vi "Navigation_Main_r1.3(new math for dist calc).vi"() -> ()   [LabVIEW 2015]
uses:
  <vilib>/myRIO/Instrument Drivers/Onboard IO/PWM/typedefs/PWM Reference.ctl
  <vilib>/myRIO/Common/Instrument Driver Framework/Utilities/typedefs/myRIO Generic Hardware Reference.ctl
  <vilib>/myRIO/Common/Instrument Driver Framework/Utilities/typedefs/Hardware Version Enum.ctl
  <vilib>/myRIO/Common/Instrument Driver Framework/Utilities/typedefs/myRIO v1.0 Reference.ctl
  <vilib>/myRIO/Common/Instrument Driver Framework/Utilities/typedefs/Generic FPGA Reference.ctl
  <vilib>/myRIO/Common/Instrument Driver Framework/myRIO v1.0/PWM/typedefs/PWM Channels Enum.ctl
  <vilib>/myRIO/Instrument Drivers/Onboard IO/PWM/typedefs/PWM Configuration.ctl
  <vilib>/userdefined/High Color/nirio_resource_hc.ctl
  <vilib>/myRIO/Common/Instrument Driver Framework/myRIO v1.0/PWM/vis/myRIO v1.1 Open PWM.vi
  <vilib>/myRIO/Common/Instrument Driver Framework/Utilities/vis/Validate Channels.vi
  <vilib>/myRIO/Common/Instrument Driver Framework/myRIO v1.0/PWM/vis/myRIO v1.0 Reserve PWM.vi
  <vilib>/myRIO/Common/Instrument Driver Framework/myRIO v1.0/PWM/vis/myRIO v1.0 Close PWM.vi
  <vilib>/myRIO/Common/Instrument Driver Framework/myRIO v1.0/PWM/vis/myRIO v1.0 Build MUX Configuration PWM.vi
  <vilib>/myRIO/Common/Instrument Driver Framework/myRIO v1.0/Resource Manager/vis/myRIO v1.0 Reserve Channel List.vi
  <vilib>/myRIO/Common/Instrument Driver Framework/myRIO v1.0/PWM/vis/myRIO v1.0 Unreserve PWM.vi
  <vilib>/myRIO/Common/Instrument Driver Framework/myRIO v1.0/Resource Manager/vis/myRIO v1.0 Create Configuration List.vi
  <vilib>/myRIO/Common/Instrument Driver Framework/myRIO v1.0/Resource Manager/vis/myRIO v1.0 Reserve Channel.vi
  <vilib>/myRIO/Common/Instrument Driver Framework/myRIO v1.0/Resource Manager/vis/myRIO v1.0 Unreserve Channel.vi
  <vilib>/myRIO/Common/Instrument Driver Framework/myRIO v1.0/Resource Manager/vis/myRIO v1.0 Unreserve Channel List.vi
  <vilib>/myRIO/Common/Instrument Driver Framework/myRIO v1.0/Resource Manager/vis/myRIO v1.0 Build Mutex Name.vi
  <vilib>/FPGAPlugInAG/myRIO-1900/niLvFpga_Open_myRIO-1900.vi
  <vilib>/rvi/interface/common/dynamic/niFpgaDynamicAddResources.vi
  <vilib>/myRIO/Common/Instrument Driver Framework/Utilities/vis/FPGA Ref Manager.vi
  <vilib>/Utility/error.llb/Error Cluster From Error Code.vi
  <vilib>/myRIO/Common/Instrument Driver Framework/Utilities/vis/Ref Counter.vi
  <vilib>/rvi/errors/niLvFpgaAdjustHostInterfaceError.vi
  <vilib>/Utility/VariantDataType/GetNumericInfo.vi
  <vilib>/myRIO/Common/Instrument Driver Framework/myRIO v1.0/myRIO v1.1 Open.vi
  <vilib>/myRIO/Common/Instrument Driver Framework/Utilities/vis/IO Manager.vi
  <vilib>/myRIO/Common/Instrument Driver Framework/Utilities/vis/Configuration Manager.vi
  <vilib>/myRIO/Common/Instrument Driver Framework/myRIO v1.0/Resource Manager/vis/myRIO v1.0 Configure IO.vi
  <vilib>/myRIO/Common/Instrument Driver Framework/myRIO v1.0/myRIO v1.0 Close.vi
  <vilib>/myRIO/Common/Instrument Driver Framework/myRIO v1.0/PWM/vis/myRIO v1.0 Write PWM.vi
  <vilib>/myRIO/Common/Instrument Driver Framework/myRIO v1.0/PWM/vis/myRIO v1.0 Shutdown PWM.vi
  <vilib>/rvi/interface/nirviOpenFPGA/nirviOpenFPGA.xnode
  Navi/E/FPGA Bitfiles/NavigationProjec_FPGATarget2_FPGAMainNavigati_PWPHW8gwDxI.lvbitx
  <vilib>/rvi/interface/nirviReadWriteControl/nirviReadWriteControl.xnode
  <vilib>/myRIO/Instrument Drivers/Onboard IO/PWM/vis/myRIO PWM Open.xnode
  <vilib>/myRIO/Instrument Drivers/Onboard IO/PWM/PWM.lvlib
  <vilib>/myRIO/Instrument Drivers/Utilities/Utilities.lvlib
  NiFpgaLv.dll
  <vilib>/rvi/interface/Simulation/niFpgaSimulationCallBeginRW.vi
panel:
  out "Tick Count(mSec) 2":u32 caption="Tick Count(mSec)"
  out "Left Setpoint":dbl
  out "Right Setpoint":dbl
  out "robot desired velocity y component\n u2 (ft/s)":dbl
  out "robot desired velocity x component\n u1 (ft/s)":dbl
  out "Desired Velocity":dbl
  out "Reset X Y":dbl
  out "Scale":dbl=1.0
  out "x traveled":dbl
  out "Omega":dbl format="%.2f"
  out "Phi desired":dbl
  out "v right wheel":dbl
  out "v left wheel":dbl
  out "max v":dbl
  in  "loc_x":dbl
  out "x delta":dbl
  out "x position camera":dbl
  out "encoder step sub vi output":dbl[](array[numeric])
  out "Avg R Dist New":dbl
  out "Avg R Step":dbl
  out "Avg L Dist New":dbl
  out "Avg L Step":dbl
  out "Distance Step":dbl
  in  "Avg R Dist Old":dbl
  in  "Avg L Dist Old":dbl
  out "encoder sub vi input array":dbl[](array[numeric])
  out "x & y position output array":dbl[](array[numeric])
  out "x & y position input array":dbl[](array[numeric])
  out "y traveled new":dbl
  out "y position":dbl
  out "x traveled new":dbl
  out "x position":dbl
  out "phi new":dbl
  in  "x traveled old":dbl
  in  "y traveled old":dbl
  in  "phi old":dbl
  in  "Phi Current":dbl format="%#_13g"
  out "omega and angular velocity calc output array":dbl[](array[numeric])
  out "omega and angular velocity calc input array":dbl[](array[numeric])
  out "Wheel  PID SetPoint input Array":dbl[](array[numeric])
  out "Wheel  PID SetPoint output Array":dbl[](array[numeric])
  in  "Goal Position Y":dbl=5.0
  out "track width(ft)":dbl=4.0
  out "RM Distance (ft)":dbl
  out "RR Distance (ft)":dbl
  out "LF Distance (ft)":dbl
  out "LM Distance (ft)":dbl
  out "RF Distance (ft)":dbl
  out "LR Distance (ft)":dbl
  in  "Start Position Y":dbl=5.0
  in  "Goal Position X":dbl=5.0
  in  "Start Position X":dbl=1.0
  in  "All Stop":bool
  in  "Left Side PID Gains":T1={"proportional gain (Kc)"=0.002, "integral time (Ti, min)"=7e-07, "derivative time (Td, min)"=0.0} {"derivative time (Td, min)" format="%.8f"; "integral time (Ti, min)" format="%.8f"; "proportional gain (Kc)" format="%.8f"}
  in  "Left Side Output Range":cluster{"output high":dbl, "output low":dbl}={"output high"=0.13333, "output low"=-0.13333} {"output low" format="%.5f"; "output high" format="%.5f"}
  in  "Right Side PID Gains":T1={"proportional gain (Kc)"=0.002, "integral time (Ti, min)"=7e-07, "derivative time (Td, min)"=0.0} {"derivative time (Td, min)" format="%.8f"; "integral time (Ti, min)" format="%.8f"; "proportional gain (Kc)" format="%.8f"}
  in  "Right Side Output Range":cluster{"output high":dbl, "output low":dbl}={"output high"=0.13333, "output low"=-0.13333} {"output low" format="%.5f"; "output high" format="%.5f"}
  out "Left PWM":dbl
  out "Right PWM":dbl
  out "LF Rot Velocity (rot/s)":dbl
  out "LM Rot Velocity (rot/s)":dbl
  out "LR Rot Velocity (rot/s)":dbl
  out "RR Rot Velocity (rot/s)":dbl
  out "RM Linear Velocity (rot/s)":dbl
  out "RF Linear Velocity (rot/s)":dbl
  in  "Encoder Reset":bool
  out "SYS.SELECTA":u8 format="%08b"
  out "ENC.B_c.CNTR":i32
  out "ENC.B_b.CNTR":i32
  out "ENC.B_a.CNTR":i32
  out "ENC.A_c.CNTR":i32
  out "ENC.A_b.CNTR":i32
  out "ENC.A_a.CNTR":i32
  out "Current Rot Velocity (rot/s)":T2(graph)
  # "Motor Control Parameters"
  # "Press Go when Start and Goal Are Set"
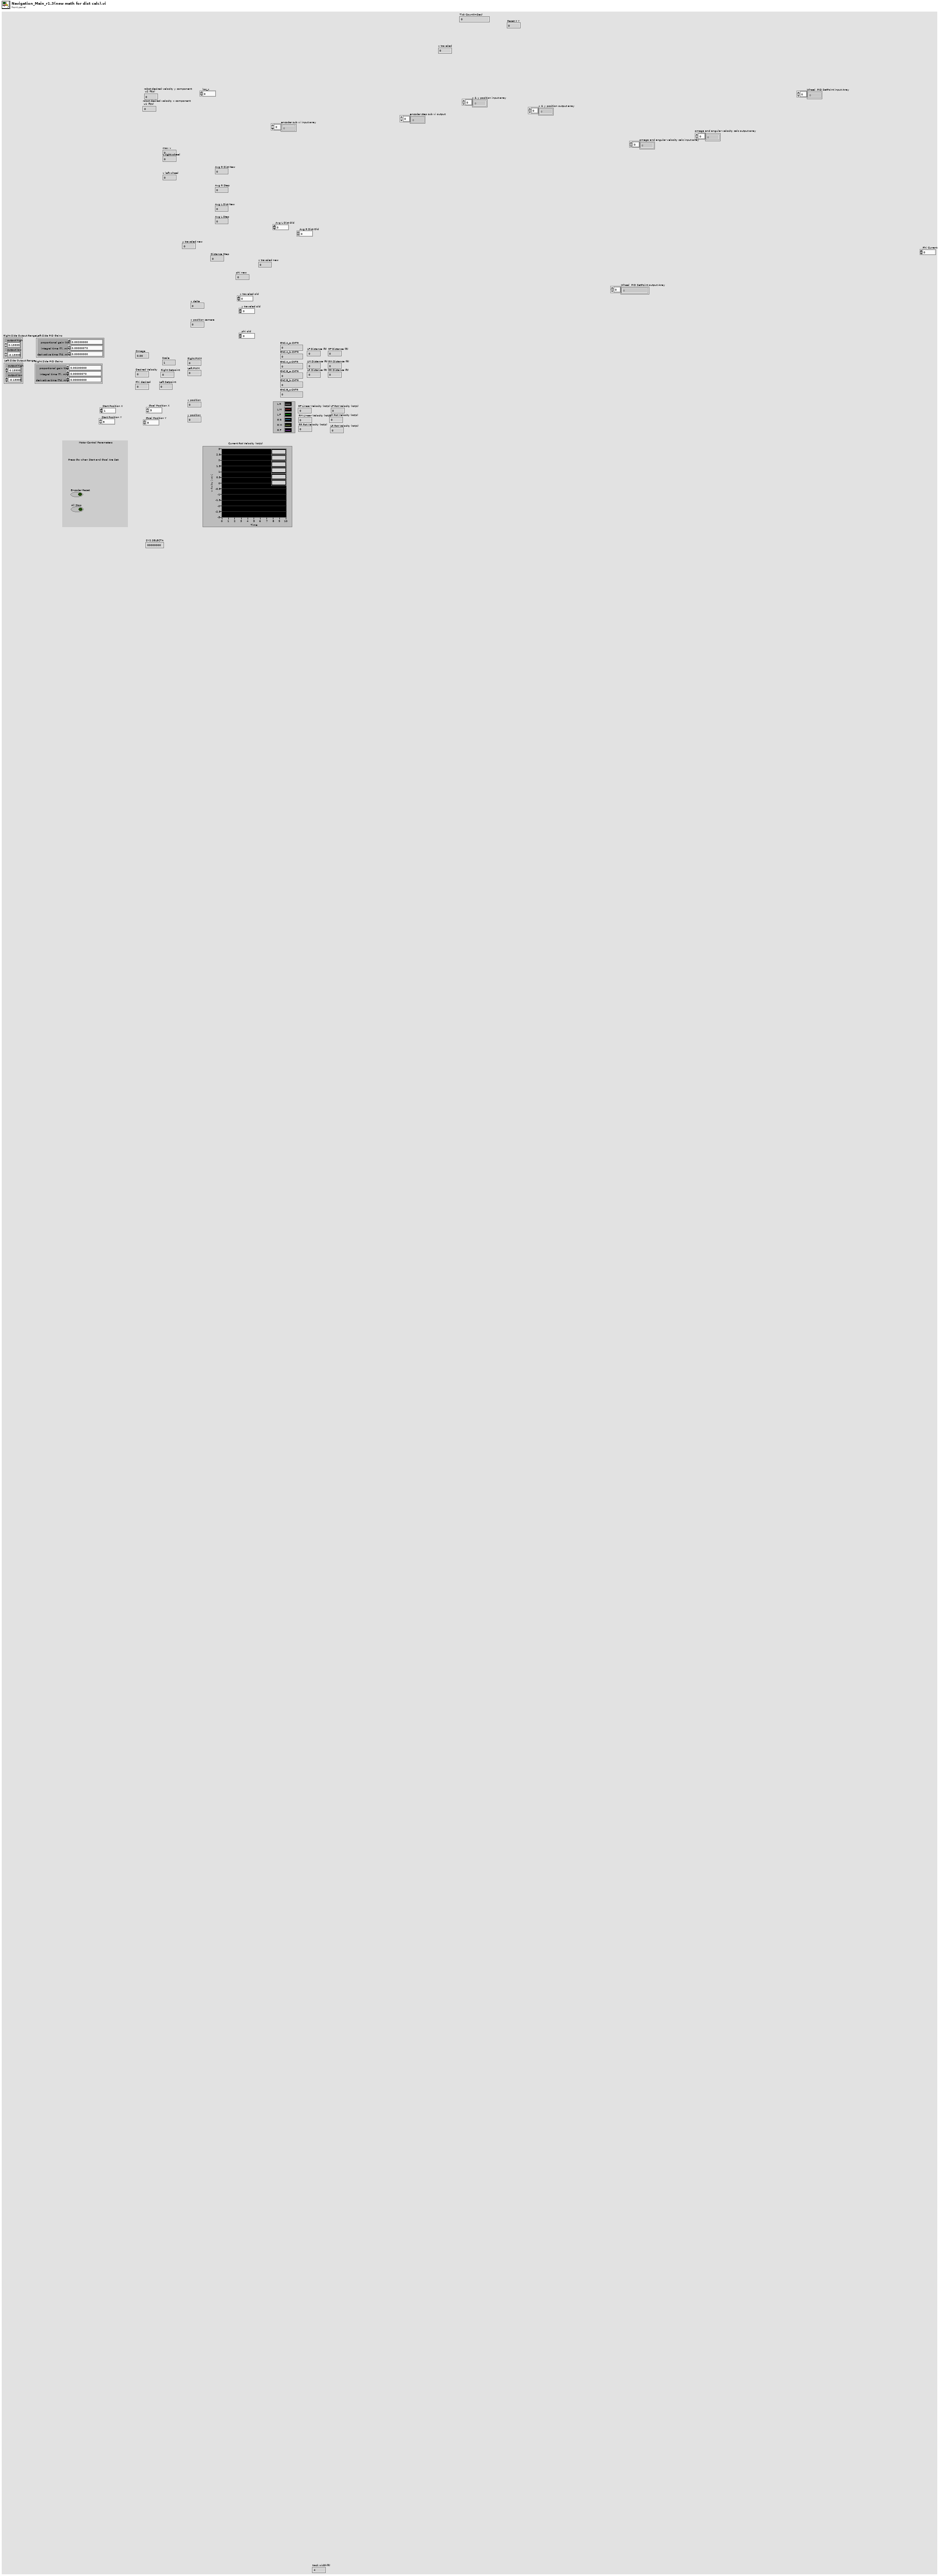
[diagram p1: front panel]
types:
  T1 = cluster{"proportional gain (Kc)":dbl, "integral time (Ti, min)":dbl, "derivative time (Td, min)":dbl}
  T2 = cluster{"Rotational Velocity (RPS)":dbl, "Rotational Velocity (RPS)":dbl, "Rotational Velocity (RPS)":dbl, "Rotational Velocity (RPS)":dbl, "Rotational Velocity (RPS)":dbl, "Rotational Velocity (RPS)":dbl}
  T3 = typedef "nirio_resource_hc.ctl" = tag
  T4 = typedef "Hardware Version Enum.ctl" = enum16{"Unknown", "myRIO-1900", "myRIO-1950", "roboRIO"}
  T5 = typedef "PWM.lvlib/PWM Reference.ctl" = cluster{"myRIO Reference":T6, "PWM Channels Enum":T9, "PWM Configuration":T10}
  T6 = typedef "myRIO Generic Hardware Reference.ctl" = cluster{"myRIO Model":T4, "myRIO Hardware Reference":T7}
  T7 = typedef "myRIO v1.0 Reference.ctl" = cluster{"Generic FPGA Reference":T8, "Allow multiple opens":bool}
  T8 = typedef "Generic FPGA Reference.ctl" = refnum<k20>
  T9 = typedef "PWM Channels Enum.ctl" = enum16{"Not Connected", "C/PWM0", "C/PWM1", "A/PWM0", "A/PWM1", "A/PWM2", "B/PWM0", "B/PWM1", "B/PWM2", "PWM/PWM0", "PWM/PWM1", "PWM/PWM2", "PWM/PWM3", "PWM/PWM4", "PWM/PWM5", "PWM/PWM6", "PWM/PWM7", "PWM/PWM8", "PWM/PWM9"}
  T10 = typedef "PWM.lvlib/PWM Configuration.ctl" = cluster{"Frequency":dbl, "Duty Cycle":dbl}
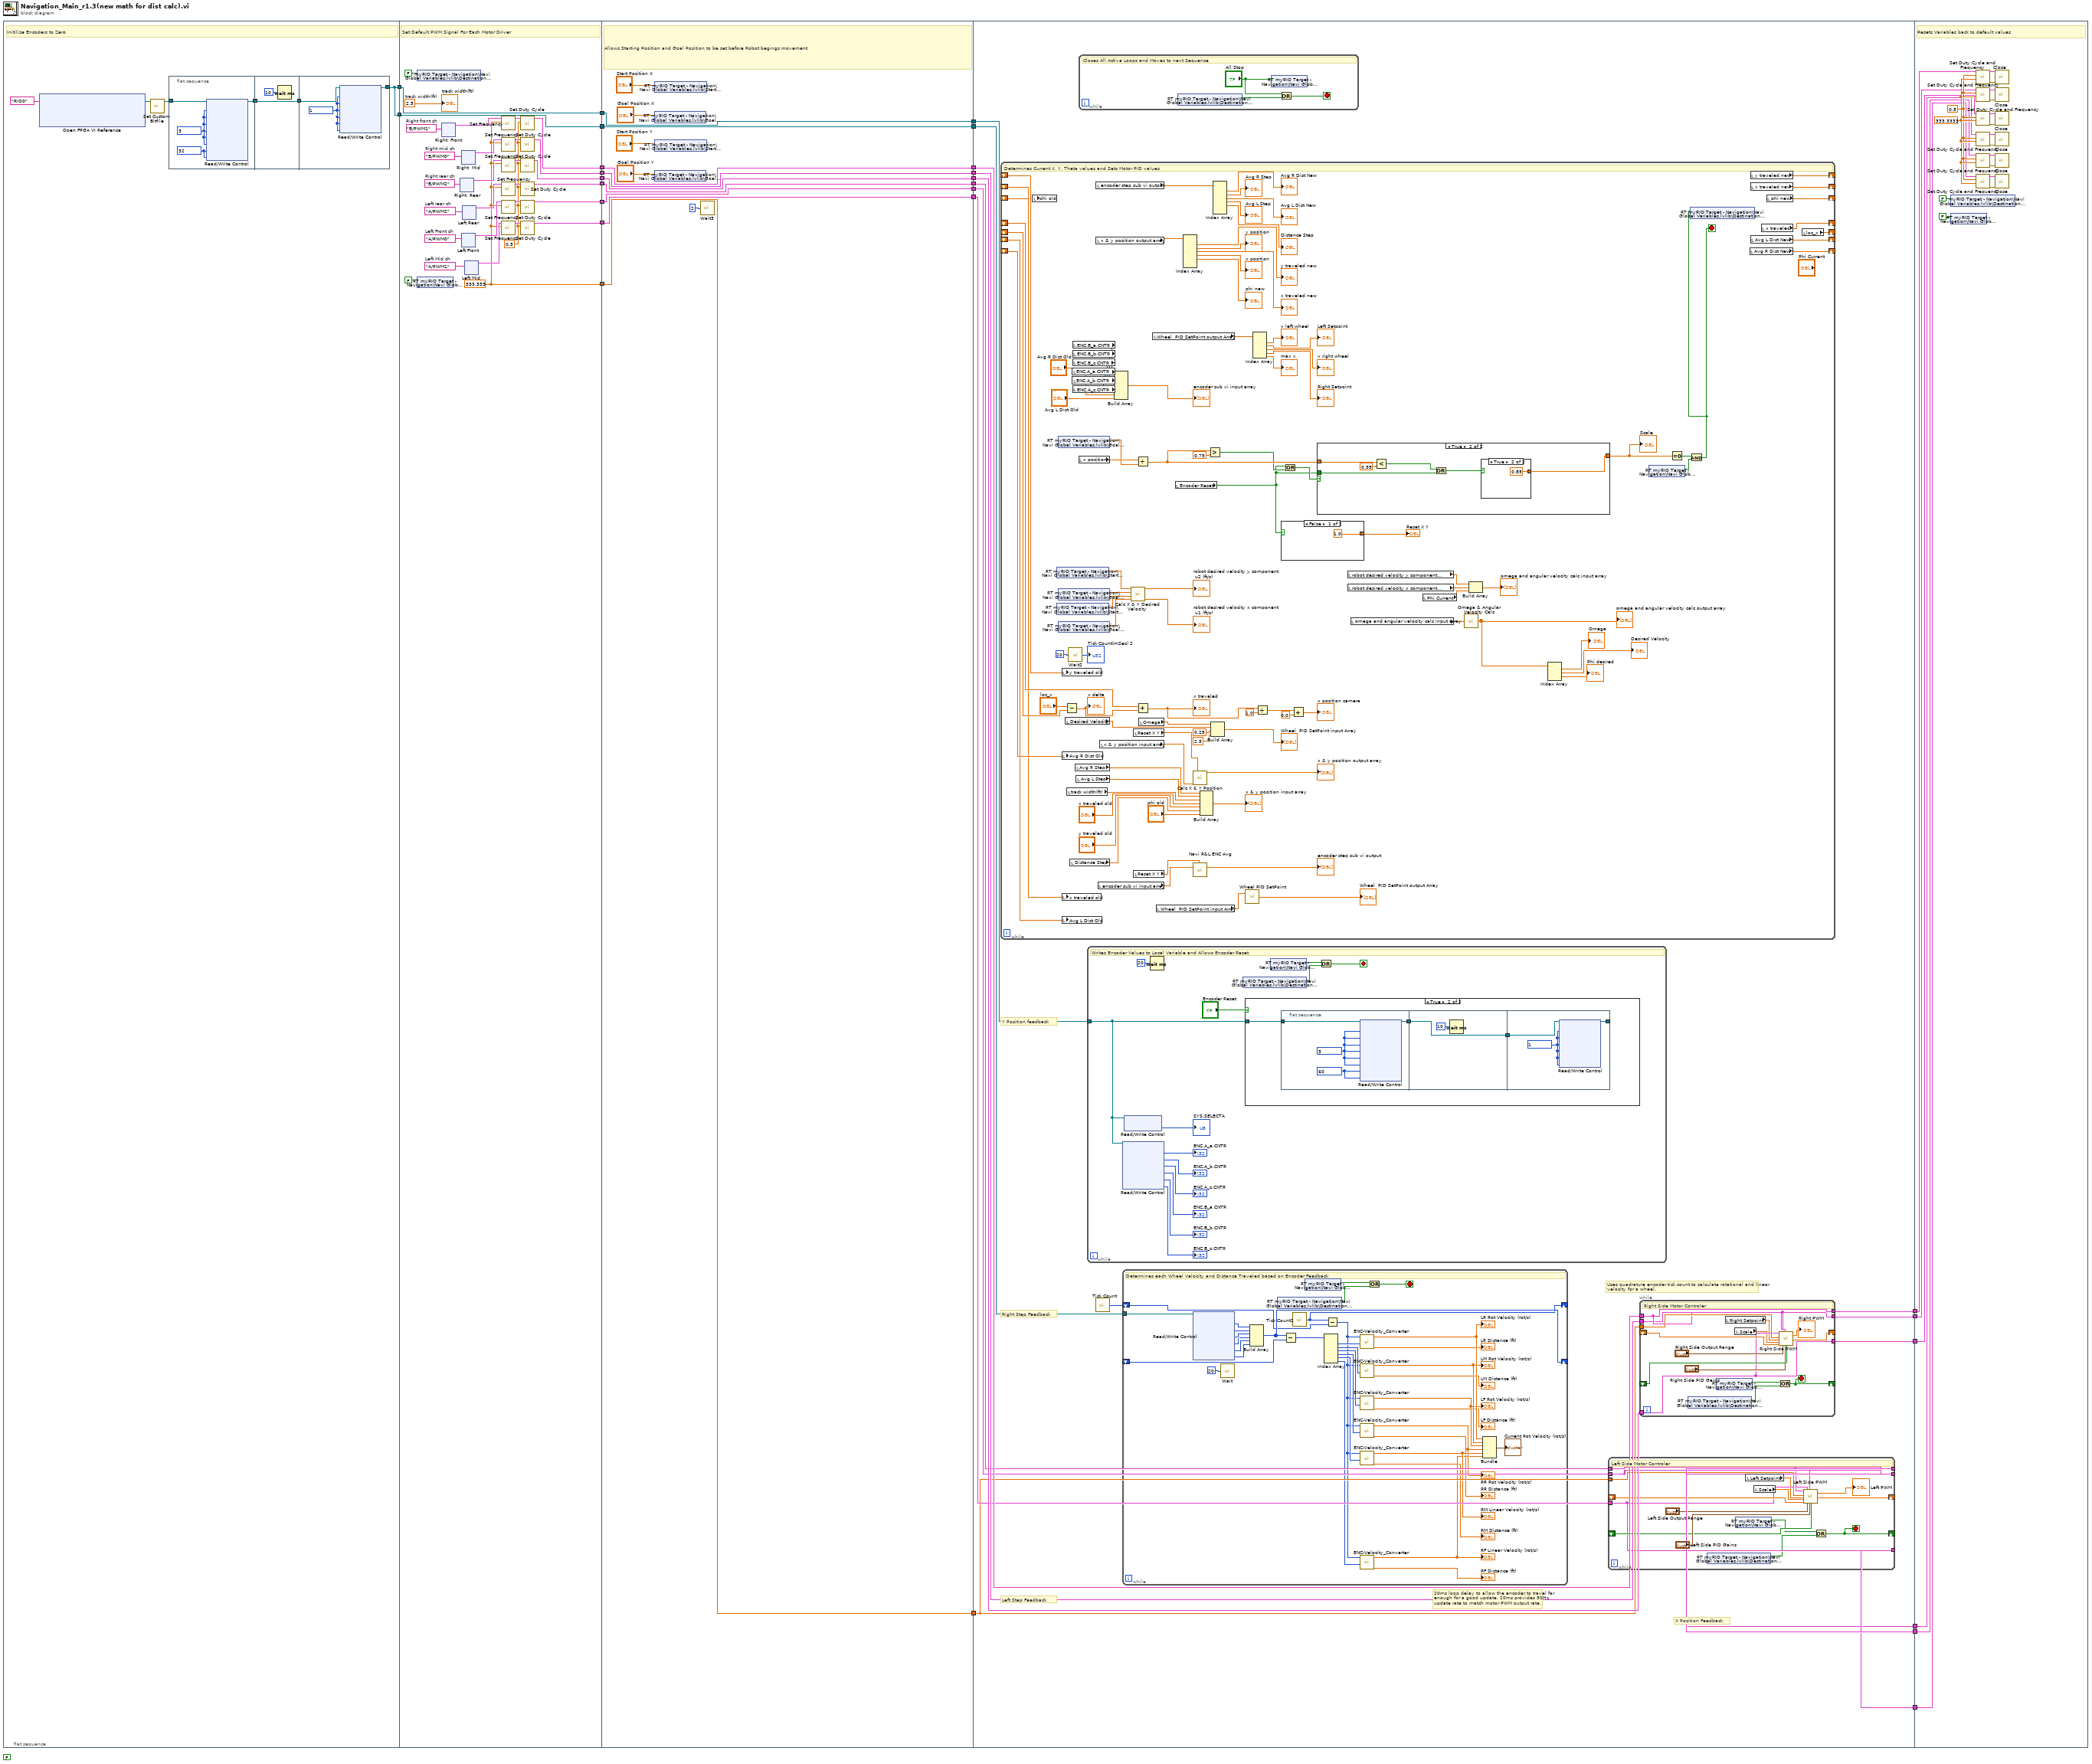
[diagram p0: block diagram]
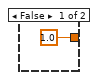
[diagram p2: hidden frame]
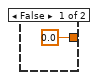
[diagram p3: hidden frame]
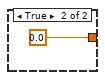
[diagram p4: hidden frame]
diagram:
  (unwired) FALSE ("stop")
  n1 = flat-sequence {
    tunnel: [w29] -> w26
    tunnel: [w29] -> w25
    tunnel: [w60] -> w24
    tunnel: [w55] -> w23
    tunnel: [w51] -> w22
    tunnel: [w50] -> w21
    tunnel: [w49] -> w20
    tunnel: [w48] -> w19
    tunnel: [w47] -> w18
    tunnel: [w46] -> w17
    tunnel: w26 -> [w45]
    tunnel: [w45] -> w16
    tunnel: w25 -> [w46]
    tunnel: w24 -> [w182]
    tunnel: [w182] -> w15
    tunnel: w23 -> [w181]
    tunnel: [w181] -> w14
    tunnel: w22 -> [w180]
    tunnel: [w180] -> w13
    tunnel: w21 -> [w169]
    tunnel: [w169] -> w12
    tunnel: w20 -> [w179]
    tunnel: [w179] -> w11
    tunnel: w19 -> [w178]
    tunnel: [w178] -> w10
    tunnel: w18 -> [w177]
    tunnel: [w177] -> w9
    tunnel: w17 -> [w176]
    tunnel: [w176] -> w8
    tunnel: w16 -> [w175]
    tunnel: [w175] -> w7
    tunnel: w15 -> [w189]
    tunnel: w14 -> [w190]
    tunnel: w13 -> [w195]
    tunnel: w12 -> [w194]
    tunnel: w11 -> [w193]
    tunnel: w10 -> [w192]
    tunnel: w9 -> [w191]
    tunnel: w8 -> [w197]
    tunnel: w7 -> [w196]
    tunnel: [w188] -> w6
    tunnel: [w187] -> w5
    tunnel: [w186] -> w4
    tunnel: [w185] -> w3
    tunnel: [w184] -> w2
    tunnel: [w183] -> w1
    tunnel: w6 -> [w409]
    tunnel: w5 -> [w408]
    tunnel: w4 -> [w407]
    tunnel: w3 -> [w406]
    tunnel: w2 -> [w405]
    tunnel: w1 -> [w404]
    frame #0 {
      # "Initilize Encoders to Zero"
      n2 = xnode "Open FPGA VI Reference"("resource name"=tag "RIO0") -> ("FPGA VI Reference Out"=w28:refnum<k20>)  [unwired: 1 in, 1 out]
      n3 = call <vilib>:"Set Custom Bitfile.vi"("Custom FPGA Reference In"=w28) -> ("Custom FPGA Reference Out"=w30:refnum<k20>)  [unwired: 9 in, 1 out]
      n4 = flat-sequence {
        tunnel: w30 -> [w35]
        tunnel: [w33] -> w32
        tunnel: w32 -> [w37]
        tunnel: [w37] -> w31
        tunnel: w31 -> [w40]
        tunnel: [w39] -> w29
        frame #0 {
          w34 = u8 32 ("SYS.SELECTA")
          w36 = u8 3 ("ENC.B_c.CNFG")
          n5 = xnode "Read/Write Control"("FPGA VI Reference In"=w35, "ENC.A_a.CNFG"=w36, "ENC.A_b.CNFG"=w36, "ENC.A_c.CNFG"=w36, "ENC.B_a.CNFG"=w36, "ENC.B_b.CNFG"=w36, "ENC.B_c.CNFG"=w36, "SYS.SELECTA"=w34, "SYS.SELECTB"=w34) -> ("FPGA VI Reference Out"=w33:refnum<k20>)  [unwired: 1 in, 1 out]
        }
        frame #1 {
          n6 = Wait (ms)(milliseconds to wait=u32 10) -> ()  [unwired: 1 out]
        }
        frame #2 {
          w41 = u8 1 ("ENC.B_c.CNFG")
          n7 = xnode "Read/Write Control"("FPGA VI Reference In"=w40, "ENC.A_a.CNFG"=w41, "ENC.A_b.CNFG"=w41, "ENC.A_c.CNFG"=w41, "ENC.B_a.CNFG"=w41, "ENC.B_b.CNFG"=w41, "ENC.B_c.CNFG"=w41) -> ("FPGA VI Reference Out"=w39:refnum<k20>)  [unwired: 1 in, 1 out]
        }
      }
    }
    frame #1 {
      w42 = 2.5  # track width(ft)
      w52 = 0.5 ("Duty Cycle")
      w60 = 333.333 ("Frequency [Hz]")
      w67 = tag "B/PWM2"  # Right rear ch
      w68 = tag "B/PWM0"  # Right mid ch
      w69 = tag "B/PWM1"  # Right front ch
      w70 = tag "A/PWM2"  # Left rear ch
      w71 = tag "A/PWM0"  # Left Front ch
      w72 = tag "A/PWM1"  # Left Mid ch
      # "Set Default PWM Signal For Each Motor Driver"
      n8 = shared-variable "RT myRIO Target - Navigation\\Navi Global Variables.lvlib\\Destination Reached"(FALSE) -> ()  [unwired: 1 in, 1 out]
      n9 = shared-variable "RT myRIO Target - Navigation\\Navi Global Variables.lvlib\\All Stop"(FALSE) -> ()  [unwired: 1 in, 1 out]
      n10 = xnode "Right  Front"("Channel Name"=w69) -> ("PWM Ref Out"=w63:T5)  [unwired: 2 in, 1 out]
      n11 = xnode "Right  Rear"("Channel Name"=w67) -> ("PWM Ref Out"=w61:T5)  [unwired: 2 in, 1 out]
      n12 = xnode "Right  Mid"("Channel Name"=w68) -> ("PWM Ref Out"=w62:T5)  [unwired: 2 in, 1 out]
      n13 = xnode "Left Front"("Channel Name"=w71) -> ("PWM Ref Out"=w65:T5)  [unwired: 2 in, 1 out]
      n14 = xnode "Left Rear"("Channel Name"=w70) -> ("PWM Ref Out"=w64:T5)  [unwired: 2 in, 1 out]
      n15 = xnode "Left Mid"("Channel Name"=w72) -> ("PWM Ref Out"=w66:T5)  [unwired: 2 in, 1 out]
      n16 = call <vilib>:"Set Frequency.vi"("Frequency [Hz]"=w60, "PWM Ref In"=w63) -> ("PWM Ref Out"=w56:T5)  [unwired: 7 in, 1 out]
      n17 = call <vilib>:"Set Frequency.vi"("Frequency [Hz]"=w60, "PWM Ref In"=w62) -> ("PWM Ref Out"=w57:T5)  [unwired: 7 in, 1 out]
      n18 = call <vilib>:"Set Frequency.vi"("Frequency [Hz]"=w60, "PWM Ref In"=w61) -> ("PWM Ref Out"=w58:T5)  [unwired: 7 in, 1 out]
      n19 = call <vilib>:"Set Frequency.vi"("Frequency [Hz]"=w60, "PWM Ref In"=w64) -> ("PWM Ref Out"=w54:T5)  [unwired: 7 in, 1 out]
      n20 = call <vilib>:"Set Frequency.vi"("Frequency [Hz]"=w60, "PWM Ref In"=w65) -> ("PWM Ref Out"=w53:T5)  [unwired: 7 in, 1 out]
      n21 = call <vilib>:"Set Frequency.vi"("Frequency [Hz]"=w60, "PWM Ref In"=w66) -> ("PWM Ref Out"=w59:T5)  [unwired: 7 in, 1 out]
      n22 = call <vilib>:"Set Duty Cycle.vi"("Duty Cycle"=w52, "PWM Ref In"=w56) -> ("PWM Ref Out"=w51:T5)  [unwired: 7 in, 1 out]
      n23 = call <vilib>:"Set Duty Cycle.vi"("Duty Cycle"=w52, "PWM Ref In"=w57) -> ("PWM Ref Out"=w50:T5)  [unwired: 7 in, 1 out]
      n24 = call <vilib>:"Set Duty Cycle.vi"("Duty Cycle"=w52, "PWM Ref In"=w58) -> ("PWM Ref Out"=w49:T5)  [unwired: 7 in, 1 out]
      n25 = call <vilib>:"Set Duty Cycle.vi"("Duty Cycle"=w52, "PWM Ref In"=w54) -> ("PWM Ref Out"=w55:T5)  [unwired: 7 in, 1 out]
      n26 = call <vilib>:"Set Duty Cycle.vi"("Duty Cycle"=w52, "PWM Ref In"=w53) -> ("PWM Ref Out"=w48:T5)  [unwired: 7 in, 1 out]
      n27 = call <vilib>:"Set Duty Cycle.vi"("Duty Cycle"=w52, "PWM Ref In"=w59) -> ("PWM Ref Out"=w47:T5)  [unwired: 7 in, 1 out]
      "track width(ft)" <- w42
    }
    frame #2 {
      # "Allows Starting Position and Goal Position to be set before Robot begings movement"
      n28 = shared-variable "RT myRIO Target - Navigation\\Navi Global Variables.lvlib\\Start Position X"("Start Position X") -> ()  [unwired: 1 in, 1 out]
      n29 = shared-variable "RT myRIO Target - Navigation\\Navi Global Variables.lvlib\\Goal Position X"("Goal Position X") -> ()  [unwired: 1 in, 1 out]
      n30 = shared-variable "RT myRIO Target - Navigation\\Navi Global Variables.lvlib\\Start Position Y"("Start Position Y") -> ()  [unwired: 1 in, 1 out]
      n31 = shared-variable "RT myRIO Target - Navigation\\Navi Global Variables.lvlib\\Goal Position Y"("Goal Position Y") -> ()  [unwired: 1 in, 1 out]
      n32 = call "Wait3"("Count(mSec)"=u32 2) -> ()  [unwired: 1 out]
    }
    frame #3 {
      # "Left Step Feedback"
      # "Y Position feedback"
      # "Right Step Feedback"
      # "X Position Feedback"
      # "Uses quadrature encoder tick count to calculate rotational and linear velocity for a wheel."
      # "20ms loop delay to allow the encoder to travel far enough for a good update. 20ms provides 50Hz update rate to match motor PWM output rate."
      n33 = while {
        shift-right: [w278] -> _
        shift-left: _ -> [w279]
        shift-right: [w275] -> _
        shift-left: _ -> [w276]
        shift-right: [w238] -> _
        shift-left: _ -> [w260]
        shift-right: [w239] -> _
        shift-left: _ -> [w261]
        shift-right: [w235] -> _
        shift-left: _ -> [w229]
        shift-right: [w236] -> _
        shift-left: _ -> [w230]
        shift-right: [w237] -> _
        shift-left: _ -> [w228]
        stop <- w200 stop-if-true
        # "Determines Current X, Y, Theta values and Sets Motor PID values"
        n34 = local write "phi old"(w228) -> ()
        n35 = shared-variable "RT myRIO Target - Navigation\\Navi Global Variables.lvlib\\Start Position Y"() -> (w293:dbl)  [unwired: 1 in, 1 out]
        n36 = shared-variable "RT myRIO Target - Navigation\\Navi Global Variables.lvlib\\Start Position X"() -> (w291:dbl)  [unwired: 1 in, 1 out]
        n37 = shared-variable "RT myRIO Target - Navigation\\Navi Global Variables.lvlib\\Goal Position X"() -> (w285:dbl)  [unwired: 1 in, 1 out]
        n38 = shared-variable "RT myRIO Target - Navigation\\Navi Global Variables.lvlib\\Goal Position Y"() -> (w292:dbl)  [unwired: 1 in, 1 out]
        n39 = shared-variable "RT myRIO Target - Navigation\\Navi Global Variables.lvlib\\Goal Position X"() -> (w290:dbl)  [unwired: 1 in, 1 out]
        n40 = local write "y traveled old"(w229) -> ()
        n41 = local write "Avg R Dist Old"(w261) -> ()
        n42 = local write "x traveled old"(w230) -> ()
        n43 = local write "Avg L Dist Old"(w260) -> ()
        n44 = Subtract(x="loc_x", y=w279) -> (x-y=w277:dbl)
        "x delta" <- w277
        n45 = local read "Desired Velocity"() -> (w217:dbl)
        n46 = local read "track width(ft)"() -> (w248:dbl)
        n47 = call "Wait2"("Count(mSec)"=u32 20) -> ("Tick Count(mSec)"=→"Tick Count(mSec) 2":u32)
        n48 = local read "Distance Step"() -> (w232:dbl)
        n49 = local read "ENC.A_a.CNTR"() -> (w254:i32)
        n50 = local read "ENC.A_b.CNTR"() -> (w255:i32)
        n51 = local read "ENC.B_a.CNTR"() -> (w251:i32)
        n52 = local read "ENC.B_b.CNTR"() -> (w252:i32)
        n53 = local read "ENC.B_c.CNTR"() -> (w253:i32)
        n54 = local read "ENC.A_c.CNTR"() -> (w256:i32)
        n55 = local read "Avg R Step"() -> (w250:dbl)
        n56 = local read "Avg L Step"() -> (w249:dbl)
        n57 = local read "x position"() -> (w204:dbl)
        n58 = local read "encoder step sub vi output"() -> (w264:dbl[])
        n59 = local read "x & y position output array"() -> (w243:dbl[])
        n60 = local read "encoder sub vi input array"() -> (w269:dbl[])
        n61 = local read "x & y position input array"() -> (w227:dbl[])
        n62 = Build Array(w251, w252, w253, w254, w255, w256, "Avg R Dist Old", "Avg L Dist Old") -> (→"encoder sub vi input array":dbl[])
        n63 = call "Calc X & Y Desired Velocity.vi"("x goal"=w290, "x start"=w291, "Y Goal"=w292, "Y Position"=w293) -> ("robot desired velocity x component\n u1 (ft/s)"=→"robot desired velocity x component\n u1 (ft/s)":dbl, "robot desired velocity y component\n u2 (ft/s)"=→"robot desired velocity y component\n u2 (ft/s)":dbl)  [unwired: 6 in]
        n64 = local read "Reset X Y"() -> (w226:dbl)
        n65 = local read "Reset X Y"() -> (w270:dbl)
        n66 = Divide(x=w204, y=w285) -> (x/y=w286:dbl)
        n67 = Add(x=w276, y=w277) -> (x+y=w274:dbl)
        "x traveled" <- w274
        n68 = local read "Omega"() -> (w216:dbl)
        n69 = local read "Wheel  PID SetPoint output Array"() -> (w210:dbl[])
        n70 = local read "Wheel  PID SetPoint input Array"() -> (w212:dbl[])
        n71 = local read "Encoder Reset"() -> (w280:bool)
        n72 = Index Array(array=w243) -> (element #1=→"y traveled new":dbl, element #2=→"y position":dbl, element #3=→"x traveled new":dbl, element #4=→"x position":dbl, element #5=→"phi new":dbl)  [unwired: 7 in, 2 out]
        n73 = call "Calc X & Y Position.vi"("x & y position input array"=w227, "Reset X Y"=w226) -> ("y & x traveled output array"=→"x & y position output array":dbl[])  [unwired: 16 in, 1 out]
        n74 = call "Navi R&L ENC Avg.vi"("encoder step sub vi input"=w269, "Reset X Y"=w270) -> ("encoder step sub vi output"=→"encoder step sub vi output":dbl[])  [unwired: 17 in]
        n75 = Build Array(w250, w249, w248, "x traveled old", "y traveled old", w232, "phi old") -> (→"x & y position input array":dbl[])
        n76 = Greater?(x=w286, y=0.75) -> (0:w281:bool)
        n77 = Build Array(w216, w217, 0.25 ("element"), 2.5 ("element")) -> (→"Wheel  PID SetPoint input Array":dbl[])
        n78 = Index Array(array=w264) -> (element #1=→"Avg R Dist New":dbl, element #2=→"Avg R Step":dbl, element #3=→"Avg L Dist New":dbl, element #4=→"Avg L Step":dbl, element #5=→"Distance Step":dbl)  [unwired: 7 in, 2 out]
        n79 = call "Wheel PID SetPoint.vi"("Wheel  PID SetPoint Input Array"=w212) -> ("Wheel  PID SetPoint output Array"=→"Wheel  PID SetPoint output Array":dbl[])  [unwired: 1 in]
        n80 = Index Array(array=w210) -> (element #1=→"v left wheel":dbl, element #2=→"Left Setpoint":dbl, element #3=→"v right wheel":dbl, element #4=→"Right Setpoint":dbl, element #5=→"max v":dbl)  [unwired: 5 in]
        n81 = Divide(x=w274, y=1.0) -> (x/y=w272:dbl)
        n82 = case shown="False" w280 {
          tunnel: [1.0 0.0] -> w287
          frame False {
          }
          frame True {
          }
        }
        "Reset X Y" <- w287
        n83 = Or(x=w280, y=w281) -> (x .or. y?=w282:bool)
        n84 = Add(x=w272, y=0.0) -> (x+y=→"x position camera":dbl)
        n85 = case shown="True" w282 {
          tunnel: w286 -> [_ w303]
          tunnel: [1.0 w300] -> w283
          tunnel: w280 -> [_ w298]
          frame False {
          }
          frame True {
            n86 = Less?(x=w303, y=0.95) -> (x < y?=w301:bool)
            n87 = Or(x=w301, y=w298) -> (x .or. y?=w299:bool)
            n88 = case shown="True" w299 {
              tunnel: [0.0 0.85] -> w300
              frame False {
              }
              frame True {
              }
            }
          }
        }
        "Scale" <- w283
        n89 = local read "robot desired velocity y component\n u2 (ft/s)"() -> (w222:dbl)
        n90 = local read "robot desired velocity x component\n u1 (ft/s)"() -> (w224:dbl)
        n91 = local read "omega and angular velocity calc input array"() -> (w225:dbl[])
        n92 = local read "Phi Current"() -> (w223:dbl)
        n93 = call "Omega & Angular Velocity Calc.vi"("omega and angular velocity calc input array"=w225) -> ("omega and angular velocity calc output array"=w199:dbl[])  [unwired: 4 in]
        "omega and angular velocity calc output array" <- w199
        n94 = Build Array(w222, w224, w223) -> (→"omega and angular velocity calc input array":dbl[])
        n95 = Index Array(array=w199) -> (element #1=→"Omega":dbl, element #2=→"Desired Velocity":dbl, element #3=→"Phi desired":dbl)  [unwired: 3 in]
        n96 = shared-variable "RT myRIO Target - Navigation\\Navi Global Variables.lvlib\\All Stop"() -> (w294:bool)  [unwired: 1 in, 1 out]
        n97 = Equal To 0?(x=w283) -> (x = 0?=w201:bool)
        n98 = And(x=w201, y=w294) -> (x .and. y?=w200:bool)
        n99 = shared-variable "RT myRIO Target - Navigation\\Navi Global Variables.lvlib\\Destination Reached"(w200) -> ()  [unwired: 1 in, 1 out]
        n100 = local read "Avg R Dist New"() -> (w239:dbl)
        n101 = local read "y traveled new"() -> (w235:dbl)
        n102 = local read "x traveled new"() -> (w236:dbl)
        n103 = local read "Avg L Dist New"() -> (w238:dbl)
        n104 = local read "x traveled"() -> (w275:dbl)
        n105 = local read "phi new"() -> (w237:dbl)
        n106 = local read "loc_x"() -> (w278:dbl)
      }
      n107 = while {
        stop <- w310 stop-if-true
        # "Closes All Active Loops and Moves to next Sequence"
        n108 = shared-variable "RT myRIO Target - Navigation\\Navi Global Variables.lvlib\\Destination Reached"() -> (w308:bool)  [unwired: 1 in, 1 out]
        n109 = shared-variable "RT myRIO Target - Navigation\\Navi Global Variables.lvlib\\All Stop"("All Stop") -> ()  [unwired: 1 in, 1 out]
        n110 = Or(x="All Stop", y=w308) -> (x .or. y?=w310:bool)
      }
      n111 = while {
        tunnel: w197 -> [w344]
        stop <- w341 stop-if-true
        # "Writes Encoder Values to Local Variable and Allows Encoder Reset"
        n112 = xnode "Read/Write Control"("FPGA VI Reference In"=w344) -> ("ENC.A_a.CNTR"=→"ENC.A_a.CNTR":u32, "ENC.A_b.CNTR"=→"ENC.A_b.CNTR":u32, "ENC.A_c.CNTR"=→"ENC.A_c.CNTR":u32, "ENC.B_a.CNTR"=→"ENC.B_a.CNTR":u32, "ENC.B_b.CNTR"=→"ENC.B_b.CNTR":u32, "ENC.B_c.CNTR"=→"ENC.B_c.CNTR":u32)  [unwired: 1 in, 2 out]
        n113 = xnode "Read/Write Control"("FPGA VI Reference In"=w344) -> ("SYS.SELECTA"=→"SYS.SELECTA":u8)  [unwired: 1 in, 2 out]
        n114 = Wait (ms)(milliseconds to wait=u32 20) -> ()  [unwired: 1 out]
        n115 = shared-variable "RT myRIO Target - Navigation\\Navi Global Variables.lvlib\\Destination Reached"() -> (w343:bool)  [unwired: 1 in, 1 out]
        n116 = case shown="True" "Encoder Reset" {
          tunnel: w344 -> [_ w354]
          frame False {
          }
          frame True {
            n117 = flat-sequence {
              tunnel: w354 -> [w359]
              tunnel: [w357] -> w356
              tunnel: w356 -> [w361]
              tunnel: [w361] -> w355
              tunnel: w355 -> [w364]
              tunnel: [w363] -> _
              frame #0 {
                w358 = u8 60 ("SYS.SELECTA")
                w360 = u8 3 ("ENC.B_c.CNFG")
                n118 = xnode "Read/Write Control"("FPGA VI Reference In"=w359, "ENC.A_a.CNFG"=w360, "ENC.A_b.CNFG"=w360, "ENC.A_c.CNFG"=w360, "ENC.B_a.CNFG"=w360, "ENC.B_b.CNFG"=w360, "ENC.B_c.CNFG"=w360, "SYS.SELECTA"=w358, "SYS.SELECTB"=w358) -> ("FPGA VI Reference Out"=w357:refnum<k20>)  [unwired: 1 in, 1 out]
              }
              frame #1 {
                n119 = Wait (ms)(milliseconds to wait=u32 10) -> ()  [unwired: 1 out]
              }
              frame #2 {
                w365 = u8 1 ("ENC.B_c.CNFG")
                n120 = xnode "Read/Write Control"("FPGA VI Reference In"=w364, "ENC.A_a.CNFG"=w365, "ENC.A_b.CNFG"=w365, "ENC.A_c.CNFG"=w365, "ENC.B_a.CNFG"=w365, "ENC.B_b.CNFG"=w365, "ENC.B_c.CNFG"=w365) -> ("FPGA VI Reference Out"=w363:refnum<k20>)  [unwired: 1 in, 1 out]
              }
            }
          }
        }
        n121 = shared-variable "RT myRIO Target - Navigation\\Navi Global Variables.lvlib\\All Stop"() -> (w342:bool)  [unwired: 1 in, 1 out]
        n122 = Or(x=w342, y=w343) -> (x .or. y?=w341:bool)
      }
      n123 = call "Tick Count"() -> ("Tick Count(uSec)"=w198:u32)
      n124 = while {
        shift-right: [w393] -> _
        shift-left: _ -> [w392]
        shift-right: [w390] -> _
        shift-left: w198 -> [w389]
        tunnel: w196 -> [w400]
        stop <- w385 stop-if-true
        # "Determines each Wheel Velocity and Distance Traveled based on Encoder Feedback"
        n125 = xnode "Read/Write Control"("FPGA VI Reference In"=w400) -> ("ENC.A_a.CNTR"=w399:u32, "ENC.A_b.CNTR"=w398:u32, "ENC.A_c.CNTR"=w397:u32, "ENC.B_a.CNTR"=w396:u32, "ENC.B_b.CNTR"=w395:u32, "ENC.B_c.CNTR"=w394:u32)  [unwired: 1 in, 2 out]
        n126 = call "Wait"("Count(mSec)"=u32 20) -> ()  [unwired: 1 out]
        n127 = Build Array(w399, w398, w397, w396, w395, w394) -> (w393:u32[])
        n128 = shared-variable "RT myRIO Target - Navigation\\Navi Global Variables.lvlib\\Destination Reached"() -> (w387:bool)  [unwired: 1 in, 1 out]
        n129 = Subtract(x=w393, y=w392) -> (x-y=w391:u32[])
        n130 = call "Tick Count2"() -> ("Tick Count(uSec)"=w390:u32)
        n131 = shared-variable "RT myRIO Target - Navigation\\Navi Global Variables.lvlib\\All Stop"() -> (w386:bool)  [unwired: 1 in, 1 out]
        n132 = Index Array(array=w391) -> (element #1=w384:u32, element #2=w381:u32, element #3=w379:u32, element #4=w377:u32, element #5=w375:u32, element #6=w372:u32)  [unwired: 6 in]
        n133 = Subtract(x=w390, y=w389) -> (x-y=w373:u32)
        n134 = call "ENC-Velocity_Converter.vi"("delta  Encoder Count"=w384, "dt (uSec)"=w373) -> ("Distance (ft)"=→"LR Distance (ft)":dbl, "Rotational Velocity (RPS)"=w383:dbl)  [unwired: 7 in, 1 out]
        "LR Rot Velocity (rot/s)" <- w383
        n135 = call "ENC-Velocity_Converter.vi"("delta  Encoder Count"=w381, "dt (uSec)"=w373) -> ("Distance (ft)"=→"LM Distance (ft)":dbl, "Rotational Velocity (RPS)"=w382:dbl)  [unwired: 7 in, 1 out]
        "LM Rot Velocity (rot/s)" <- w382
        n136 = call "ENC-Velocity_Converter.vi"("delta  Encoder Count"=w379, "dt (uSec)"=w373) -> ("Distance (ft)"=→"LF Distance (ft)":dbl, "Rotational Velocity (RPS)"=w380:dbl)  [unwired: 7 in, 1 out]
        "LF Rot Velocity (rot/s)" <- w380
        n137 = call "ENC-Velocity_Converter.vi"("delta  Encoder Count"=w377, "dt (uSec)"=w373) -> ("Distance (ft)"=→"RR Distance (ft)":dbl, "Rotational Velocity (RPS)"=w378:dbl)  [unwired: 7 in, 1 out]
        "RR Rot Velocity (rot/s)" <- w378
        n138 = call "ENC-Velocity_Converter.vi"("delta  Encoder Count"=w375, "dt (uSec)"=w373) -> ("Distance (ft)"=→"RM Distance (ft)":dbl, "Rotational Velocity (RPS)"=w376:dbl)  [unwired: 7 in, 1 out]
        "RM Linear Velocity (rot/s)" <- w376
        n139 = call "ENC-Velocity_Converter.vi"("delta  Encoder Count"=w372, "dt (uSec)"=w373) -> ("Distance (ft)"=→"RF Distance (ft)":dbl, "Rotational Velocity (RPS)"=w374:dbl)  [unwired: 7 in, 1 out]
        "RF Linear Velocity (rot/s)" <- w374
        n140 = Or(x=w386, y=w387) -> (x .or. y?=w385:bool)
        n141 = Bundle("Rotational Velocity (RPS)"=w383, "Rotational Velocity (RPS)"=w382, "Rotational Velocity (RPS)"=w380, "Rotational Velocity (RPS)"=w378, "Rotational Velocity (RPS)"=w376, "Rotational Velocity (RPS)"=w374) -> (→"Current Rot Velocity (rot/s)":T2)  [unwired: 1 in]
      }
      n142 = while {
        tunnel: w192 -> [w318]
        tunnel: w191 -> [w317]
        tunnel: w190 -> [w316]
        tunnel: w189 -> [w325]
        shift-right: [w321] -> _
        shift-left: _ -> [w320]
        shift-right: [w313] -> _
        shift-left: _ -> [w319]
        tunnel: [w318] -> w185
        tunnel: [w317] -> w184
        tunnel: [w316] -> w183
        stop <- w313 stop-if-true
        # "Left Side Motor Controler"
        n143 = shared-variable "RT myRIO Target - Navigation\\Navi Global Variables.lvlib\\Destination Reached"() -> (w315:bool)  [unwired: 1 in, 1 out]
        n144 = shared-variable "RT myRIO Target - Navigation\\Navi Global Variables.lvlib\\All Stop"() -> (w314:bool)  [unwired: 1 in, 1 out]
        n145 = local read "Left Setpoint"() -> (w312:dbl)
        n146 = local read "Scale"() -> (w311:dbl)
        n147 = call "Left Side PWM.vi"("Left rear"=w316, "Frequency"=w325, "Left Side Setpoint"=w312, "Left Side Scale"=w311, "Left PID Feedback"=w320, "Left Mid"=w317, "Left Side Output Range"="Left Side Output Range", "Left Front"=w318, "Left Side PID Gains"="Left Side PID Gains", "Reset Left E.T."=w319) -> ("Left PWM"=→"Left PWM":dbl, "Left PID Output"=w321:dbl)  [unwired: 8 in]
        n148 = Or(x=w314, y=w315) -> (x .or. y?=w313:bool)
      }
      n149 = while {
        tunnel: w195 -> [w333]
        tunnel: w194 -> [w332]
        tunnel: w193 -> [w331]
        tunnel: w189 -> [w340]
        shift-right: [w336] -> _
        shift-left: _ -> [w335]
        shift-right: [w328] -> _
        shift-left: _ -> [w334]
        tunnel: [w333] -> w188
        tunnel: [w332] -> w187
        tunnel: [w331] -> w186
        stop <- w328 stop-if-true
        # "Right Side Motor Controler"
        n150 = shared-variable "RT myRIO Target - Navigation\\Navi Global Variables.lvlib\\Destination Reached"() -> (w330:bool)  [unwired: 1 in, 1 out]
        n151 = shared-variable "RT myRIO Target - Navigation\\Navi Global Variables.lvlib\\All Stop"() -> (w329:bool)  [unwired: 1 in, 1 out]
        n152 = local read "Right Setpoint"() -> (w327:dbl)
        n153 = local read "Scale"() -> (w326:dbl)
        n154 = Or(x=w329, y=w330) -> (x .or. y?=w328:bool)
        n155 = call "Right Side PWM.vi"("Right rear"=w331, "Frequency"=w340, "Right Side Setpoint"=w327, "Right Side Scale"=w326, "Right PID Feedback"=w335, "Right Mid"=w332, "Right Side Output Range"="Right Side Output Range", "Right Front"=w333, "Right Side PID Gains"="Right Side PID Gains", "Reset Right E.T."=w334) -> ("Right PWM"=→"Right PWM":dbl, "Right PID Output"=w336:dbl)  [unwired: 8 in]
      }
    }
    frame #4 {
      w410 = 0.5
      w411 = 333.3333
      # "Resets Variables back to default values"
      n156 = shared-variable "RT myRIO Target - Navigation\\Navi Global Variables.lvlib\\Destination Reached"(FALSE) -> ()  [unwired: 1 in, 1 out]
      n157 = shared-variable "RT myRIO Target - Navigation\\Navi Global Variables.lvlib\\All Stop"(FALSE) -> ()  [unwired: 1 in, 1 out]
      n158 = call <vilib>:"Set Duty Cycle and Frequency.vi"("Frequency [Hz]"=w411, "Duty Cycle"=w410, "PWM Ref In"=w409) -> ("error out"=w416:errorcluster, "PWM Ref Out"=w423:T5)  [unwired: 6 in]
      n159 = call <vilib>:"Set Duty Cycle and Frequency.vi"("Frequency [Hz]"=w411, "Duty Cycle"=w410, "PWM Ref In"=w408) -> ("error out"=w421:errorcluster, "PWM Ref Out"=w422:T5)  [unwired: 6 in]
      n160 = call <vilib>:"Set Duty Cycle and Frequency.vi"("Frequency [Hz]"=w411, "Duty Cycle"=w410, "PWM Ref In"=w407) -> ("error out"=w415:errorcluster, "PWM Ref Out"=w420:T5)  [unwired: 6 in]
      n161 = call <vilib>:"Set Duty Cycle and Frequency.vi"("Frequency [Hz]"=w411, "Duty Cycle"=w410, "PWM Ref In"=w404) -> ("error out"=w412:errorcluster, "PWM Ref Out"=w417:T5)  [unwired: 6 in]
      n162 = call <vilib>:"Set Duty Cycle and Frequency.vi"("Frequency [Hz]"=w411, "Duty Cycle"=w410, "PWM Ref In"=w406) -> ("error out"=w414:errorcluster, "PWM Ref Out"=w419:T5)  [unwired: 6 in]
      n163 = call <vilib>:"Set Duty Cycle and Frequency.vi"("Frequency [Hz]"=w411, "Duty Cycle"=w410, "PWM Ref In"=w405) -> ("error out"=w413:errorcluster, "PWM Ref Out"=w418:T5)  [unwired: 6 in]
      n164 = call <vilib>:"Close.vi"("error in (no error)"=w416, "PWM Ref In"=w423) -> ()  [unwired: 9 in, 1 out]
      n165 = call <vilib>:"Close.vi"("error in (no error)"=w421, "PWM Ref In"=w422) -> ()  [unwired: 9 in, 1 out]
      n166 = call <vilib>:"Close.vi"("error in (no error)"=w415, "PWM Ref In"=w420) -> ()  [unwired: 9 in, 1 out]
      n167 = call <vilib>:"Close.vi"("error in (no error)"=w412, "PWM Ref In"=w417) -> ()  [unwired: 9 in, 1 out]
      n168 = call <vilib>:"Close.vi"("error in (no error)"=w414, "PWM Ref In"=w419) -> ()  [unwired: 9 in, 1 out]
      n169 = call <vilib>:"Close.vi"("error in (no error)"=w413, "PWM Ref In"=w418) -> ()  [unwired: 9 in, 1 out]
    }
  }
